vi "Ch3_WaveformSimulator.vi"() -> ()   [LabVIEW 2015]
uses:
  <vilib>/imath/engines/lvmath2/RunTimeEngine/Managers/WorkSpace/UID Generator.vi
  <vilib>/imath/engines/lvmath2/RunTimeEngine/RunTimeType/NIMS_RunTimeType_From StrictType (excl LVString).vi
  <instcachedir>/0/NIMS_RunTimeType_From StrictType (excl LVString)_EB1C38A9BC5048DA9ABDA8F781E54D21.lvgen/NIMS_RunTimeType_From StrictType (excl LVString)_EB1C38A9BC5048DA9ABDA8F781E54D21_000.vi
  <vilib>/imath/engines/lvmath2/RunTimeEngine/LocalVariableDefStatement/MC_LocalVariableDefStatement_Display.vi
  <vilib>/imath/engines/lvmath2/RunTimeEngine/RangeToken/NIMS_Range.vi
  <instcachedir>/0/NIMS_Range_D919CC09935940E88F755EC1C6F49AC1.lvgen/NIMS_Range_D919CC09935940E88F755EC1C6F49AC1_000.vi
  <vilib>/imathl/engines/lvmath/Functions/Error Handling/Create Error.vi
  <vilib>/imath/engines/lvmath2/RunTimeEngine/Managers/SymbolTable/Clear UID.vi
  <vilib>/imath/engines/lvmath2/RunTimeEngine/NodeEndStatement/NIMS_NodeEndStatement_Output.vi
  <instcachedir>/0/NIMS_NodeEndStatement_Output_53EC0D466D134D7ABD903AC30B43404B.lvgen/NIMS_NodeEndStatement_Output_53EC0D466D134D7ABD903AC30B43404B_005.vi
  <vilib>/imath/engines/lvmath2/RunTimeEngine/ErrorHandling/NIMS_Finalize Error.vi
  <vilib>/imath/engines/lvmath2/RunTimeEngine/Managers/SymbolTable/NIMS_WorkSpace.lvlib
panel:
  in  "Shape":enum16{""}(ring)
  out "Displacement":dbl[](array[numeric])
  out "Time":dbl[](array[numeric])
  in  "Amplitude":dbl
  in  "Frequency":dbl
  in  "Sampling Frequency":dbl
  in  "Number of Samples":i32
  out "XY Graph":cluster{"t":dbl[], "x":dbl[]}(graph)
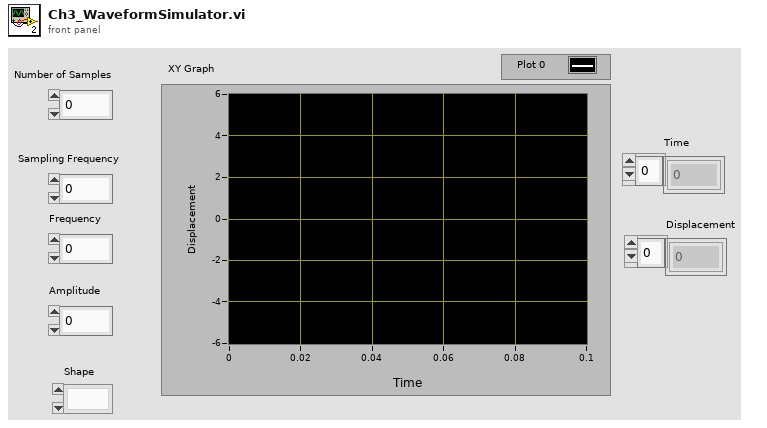
[diagram p1: front panel]
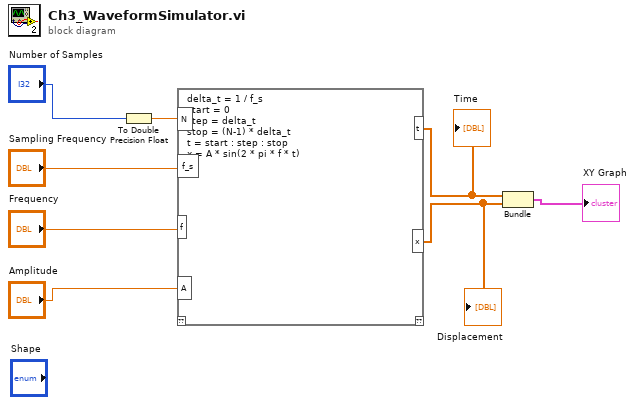
[diagram p0: block diagram]
diagram:
  n1 = To Double Precision Float(number="Number of Samples") -> (double precision float=w4:dbl)
  n2 = mathscript code="delta_t = 1 / f_s\nstart = 0\nstep = delta_t\nstop = (N-1) * delta_t\nt = start : step : stop\nx = A * sin(2 * pi * f * t)"("N"=w4, "f_s"="Sampling Frequency", "f"="Frequency", "A"="Amplitude") -> ("t"=w3:dbl[], "x"=w2:dbl[])  [unwired: 1 in, 1 out]
  "Time" <- w3
  "Displacement" <- w2
  n3 = Bundle("t"=w3, "x"=w2) -> (→"XY Graph":cluster{"t":dbl[], "x":dbl[]})  [unwired: 1 in]
